vi "Exemple_Metrics_Classification_Report.vi"() -> ()   [LabVIEW 2020]
uses:
  Objet/3 - Model selection and evaluation/3.3 - Metrics and scoring/classification_report/Classification_Report.vi
panel:
  out "String Data":string
  out "error out":errorcluster caption="sortie d'erreur"
  in  "classification_report":T1={"labels"=[], "target_names"=["C0", "C1", "C2"], "sample_weight"=[], "digits"=2, "zero_division"={"dtype_zero_division"="str", "zero_division"="warn"}}
  in  "error in (no error)":errorcluster caption="entrée d'erreur (pas d'erreur)"
  in  "y_pred":string[][](array[string])=[["0"], ["0"], ["2"], ["2"], ["1"]]
  in  "y_true":string[][](array[string])=[["0"], ["1"], ["2"], ["2"], ["2"]]
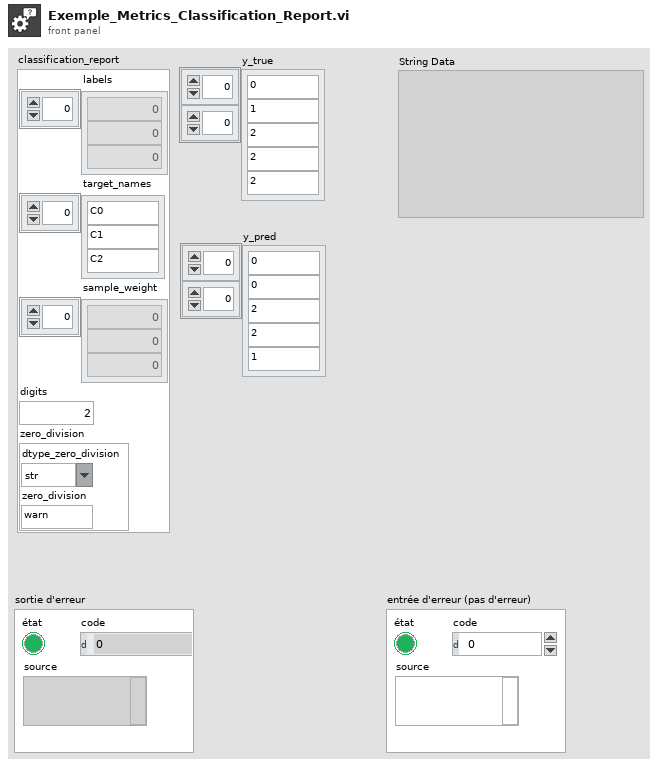
[diagram p1: front panel]
types:
  T1 = cluster{"labels":i32[], "target_names":string[], "sample_weight":dbl[], "digits":i32, "zero_division":cluster{"dtype_zero_division":string, "zero_division":string}}
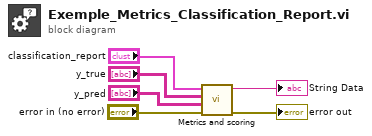
[diagram p0: block diagram]
diagram:
  n1 = call-poly "Metrics and scoring.vi"("error in (no error)"="error in (no error)", "y_pred"="y_pred", "y_true"="y_true", "classification_report"="classification_report") -> ("error out"=→"error out":errorcluster, "String Data"=→"String Data":string)  [unwired: 6 in]
